vi "SendDataCommand.vi"(8 "error in (no error)":errorcluster, 9 "Data 2":dbl[](array[numeric]), 10 "Data":dbl[](array[numeric]), 11 "Queue in":refnum<queue>) -> (0 "error out":errorcluster, 3 "Queue out":refnum<queue>)   [LabVIEW 2016]
doc: "sends the sensor data to the data analyzer loop"
uses:
  DataType.ctl
  data_command_enum.ctl
  sensor_data.ctl
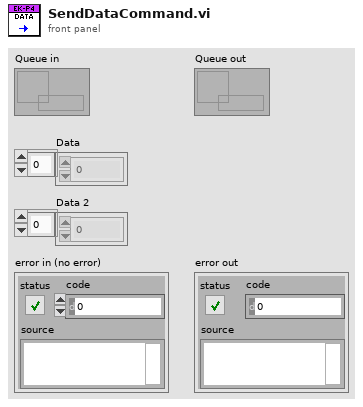
[diagram p1: front panel]
types:
  T1 = typedef "sensor_data.ctl" = cluster{"Data":dbl[], "Data 2":dbl[]}
  T2 = typedef "data_command_enum.ctl" = enum16{"data", "display", "quit", "save", "filepath", "weak left", "state", "weak right", "strong left", "strong right", "stopRecording", "close", "sid"}
  T3 = typedef "DataType.ctl" = cluster{"command":T2, "data":variant}
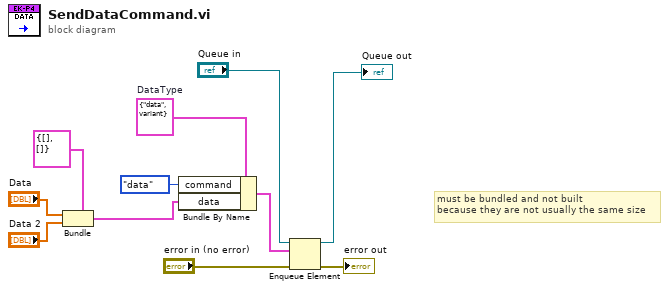
[diagram p0: block diagram]
diagram:
  w8 = T3 {"command"=enum."data", "data"=variant(dbl[] [])}  # DataType
  # "must be bundled and not built\nbecause they are not usually the same size"
  n1 = Bundle(cluster=T1 {"Data"=[], "Data 2"=[]} ("sensor data"), "Data"="Data", "Data 2"="Data 2") -> (w3:T1)
  n2 = Bundle By Name(cluster=w8, "command"=data_command_enum."data", "data"=w3) -> (w7:T3)
  n3 = Enqueue Element(queue="Queue in", element=w7, error in (no error)="error in (no error)") -> (queue out=→"Queue out":refnum<queue>, error out=→"error out":errorcluster)  [unwired: 1 in, 1 out]
